vi "Get Config.vi"(8 "error in (no error)":errorcluster, 11 "CAP-USB-1 in":refnum<class "CAP-USB-1.lvclass">) -> (0 "error out":errorcluster, 1 "Config Data":variant, 3 "CAP-USB-1 out":refnum<class "CAP-USB-1.lvclass">)   [LabVIEW 2014, in "CAP-USB-1.lvlib" / "CAP-USB-1.lvclass"]
uses:
  CAP-USB-1.lvclass
  CAP-USB-1.lvclass/CAP-USB-1.ctl
  DriverMasterSync/build/DriverMasterSync.lvlibp/Modules/HAL/DriverMasterSync/DriverMasterSyncClass/DriverMasterSync.lvclass
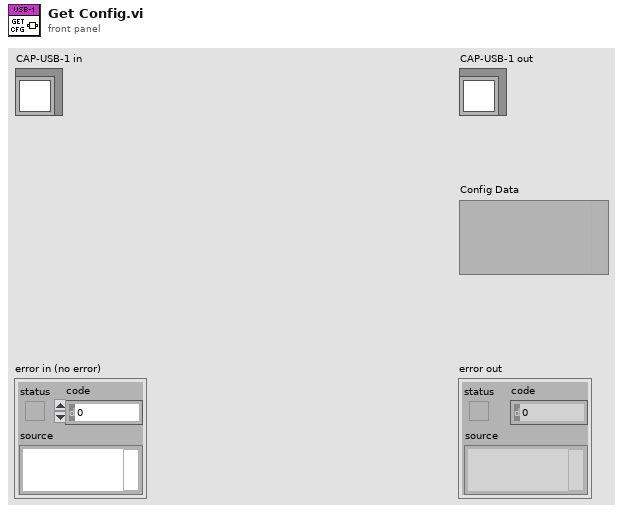
[diagram p1: front panel]
types:
  T1 = typedef "DriverMasterSync.lvlibp/HAL Config Data.ctl" = cluster{"HWSync Index":u32, "Driver Name":string, "Channel Mask":u64}
  T2 = cluster{"VISA resource name":refnum<visa-resource-name>}
  T3 = cluster{"Transductores":u64, "Delay uS":i32, "Delay uS Seq":i32, "Num de tramas":u32, "Tamaño Script":i32, "Orden Transd":u64, "Pulsos encoder":u16, "Offset":sgl[], "Gain":sgl[], "Reduccion":sgl, "Proteccion T":u64}
  T4 = cluster{"Promedio Transd":sgl[], "Tolerancia":sgl, "Test Ok":bool[], "Muestras Diag. Cycle":u32, "Tolerancia Cycle":sgl}
  T5 = cluster{"HWSync Index":u32, "Connection Data":cluster{"VISA resource name":refnum<visa-resource-name>}, "Config Data":cluster{"Transductores":u64, "Delay uS":i32, "Delay uS Seq":i32, "Num de tramas":u32, "Tamaño Script":i32, "Orden Transd":u64, "Pulsos encoder":u16, "Offset":sgl[], "Gain":sgl[], "Reduccion":sgl, "Proteccion T":u64}, "Diagnostic Data":cluster{"Promedio Transd":sgl[], "Tolerancia":sgl, "Test Ok":bool[], "Muestras Diag. Cycle":u32, "Tolerancia Cycle":sgl}, "Comandos":cluster{"Salidas":bool[]}}
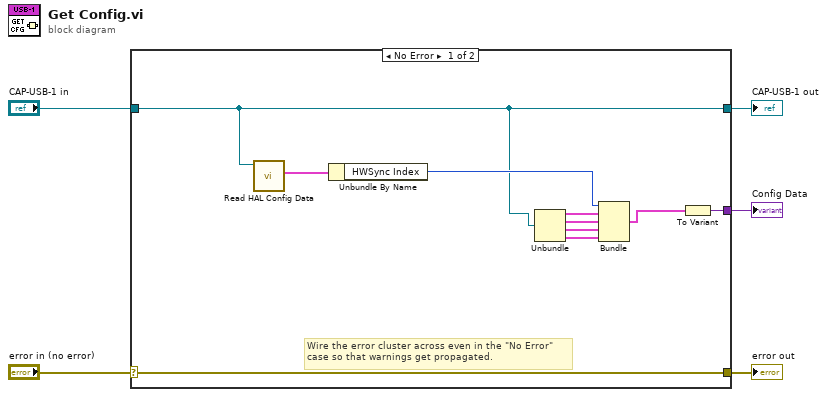
[diagram p0: block diagram]
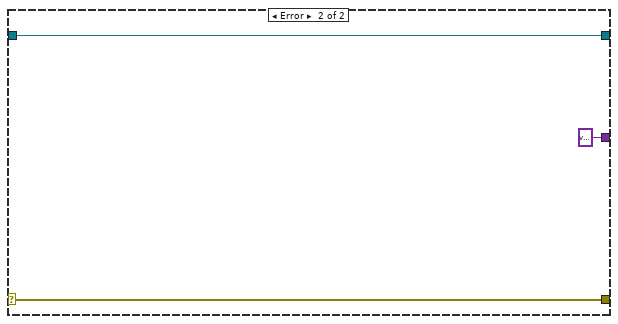
[diagram p2: hidden frame]
diagram:
  n1 = case shown="No Error" "error in (no error)" {
    selector: "error in (no error)" -> [w15 w18]
    tunnel: [w15 w18] -> w4
    tunnel: [w11 w17] -> w2
    tunnel: "CAP-USB-1 in" -> [w11 w17]
    tunnel: [w14 variant ("Variant")] -> w1
    frame No Error {
      # "Wire the error cluster across even in the \"No Error\"\ncase so that warnings get propagated."
      n2 = call "Read HAL Config Data.vi"("DriverMasterSync in"=w11) -> ("HAL Config Data"=w13:T1)  [unwired: 8 in, 2 out]
      n3 = Unbundle By Name(w13) -> ("HWSync Index"=w12:u32)
      n4 = Unbundle(w11) -> (w10:T2, w9:T3, w8:T4, w7:cluster{"Salidas":bool[]})
      n5 = Bundle("HWSync Index"=w12, "Connection Data"=w10, "Config Data"=w9, "Diagnostic Data"=w8, "Comandos"=w7) -> (w6:T5)  [unwired: 1 in]
      n6 = To Variant(anything=w6) -> (Variant=w14:variant)
    }
    frame Error {
    }
  }
  "error out" <- w4
  "CAP-USB-1 out" <- w2
  "Config Data" <- w1
